vi "table column metadata.vi"(0 "db":dbl, 1 "zDbName":string, 2 "zTableName":string, 3 "zColumnName":string, 4 "pzDataType":string, 5 "pzCollSeq":string, 6 "pNotNull":i32, 7 "error in (no error)":errorcluster, 8 "pPrimaryKey":i32, 9 "pAutoinc":i32) -> (18 "pPrimaryKey out":i32, 19 "pAutoinc out":i32, 20 "db out":dbl, 21 "function return":i32, 26 "pNotNull out":i32, 27 "error out":errorcluster)   [LabVIEW 2020, in "sqlite3.lvlib"]
uses:
  sqlite3.lvlib
  errstr.vi
  bin/sqlite3_64.dll
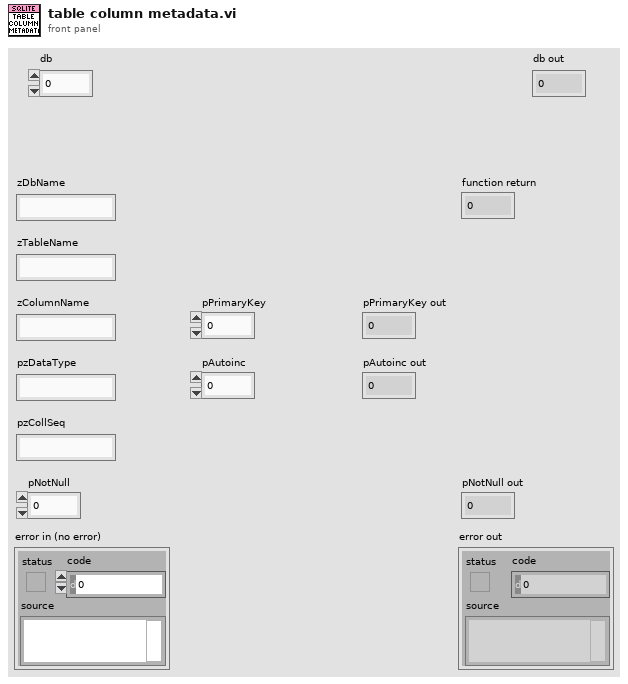
[diagram p1: front panel]
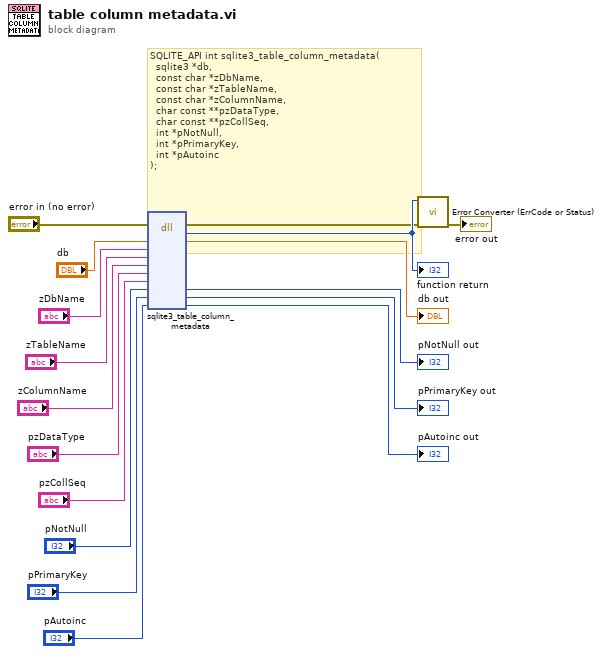
[diagram p0: block diagram]
diagram:
  # "SQLITE_API int sqlite3_table_column_metadata(\n  sqlite3 *db,                \n  const char *zDbName,        \n  const char *zTableName,     \n  const char *zColumnName,    \n  char const **pzDataType,    \n  char const **pzCollSeq,     \n  int *pNotNull,              \n  int *pPrimaryKey,           \n  int *pAutoinc               \n);"
  n1 = dll-call lib="C:/Users/Fred.Guo/Desktop/Database-configuration/externals/sqlite3/Source/bin/sqlite3_*.*" fn="sqlite3_table_column_metadata"(error in="error in (no error)", "db"="db", "zDbName"="zDbName", "zTableName"="zTableName", "zColumnName"="zColumnName", "pzDataType"="pzDataType", "pzCollSeq"="pzCollSeq", "pNotNull"="pNotNull", "pPrimaryKey"="pPrimaryKey", "pAutoinc"="pAutoinc") -> (error out=w2:errorcluster, w17:i32, "db"=→"db out":dbl, "pNotNull"=→"pNotNull out":i32, "pPrimaryKey"=→"pPrimaryKey out":i32, "pAutoinc"=→"pAutoinc out":i32)  [unwired: 7 in, 1 out]
  "function return" <- w17
  n2 = call "Error Converter (ErrCode or Status).vi"("error in (no error)"=w2, "error code"=w17) -> ("error out"=→"error out":errorcluster)  [unwired: 9 in]
